vi "HW_Server.vi"(8 "Error In":errorcluster) -> (0 "Error Out":errorcluster)   [LabVIEW 2011]
doc: "This VI will handle communication with Main VI and HW."
uses:
  Controls/TransparencyEffectOperations.ctl
  Controls/Global Stop - Operations.ctl
panel:
  # "HW SERVER"
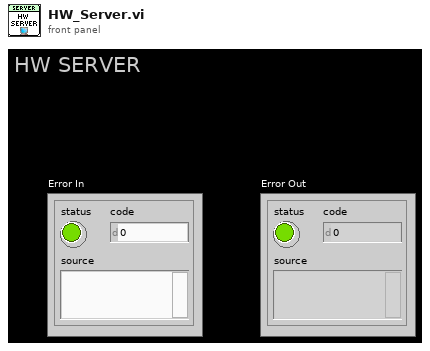
[diagram p1: front panel]
types:
  T1 = typedef "TransparencyEffectOperations.ctl" = enum16{"Show", "Hide 80%", "Hide All"}
  T2 = typedef "Global Stop - Operations.ctl" = enum16{"Stop", "Status", "Init"}
  T3 = typedef "HW Server Status.ctl" = enum16{"NO CHASSIS", "NO MODULES", "OK"}
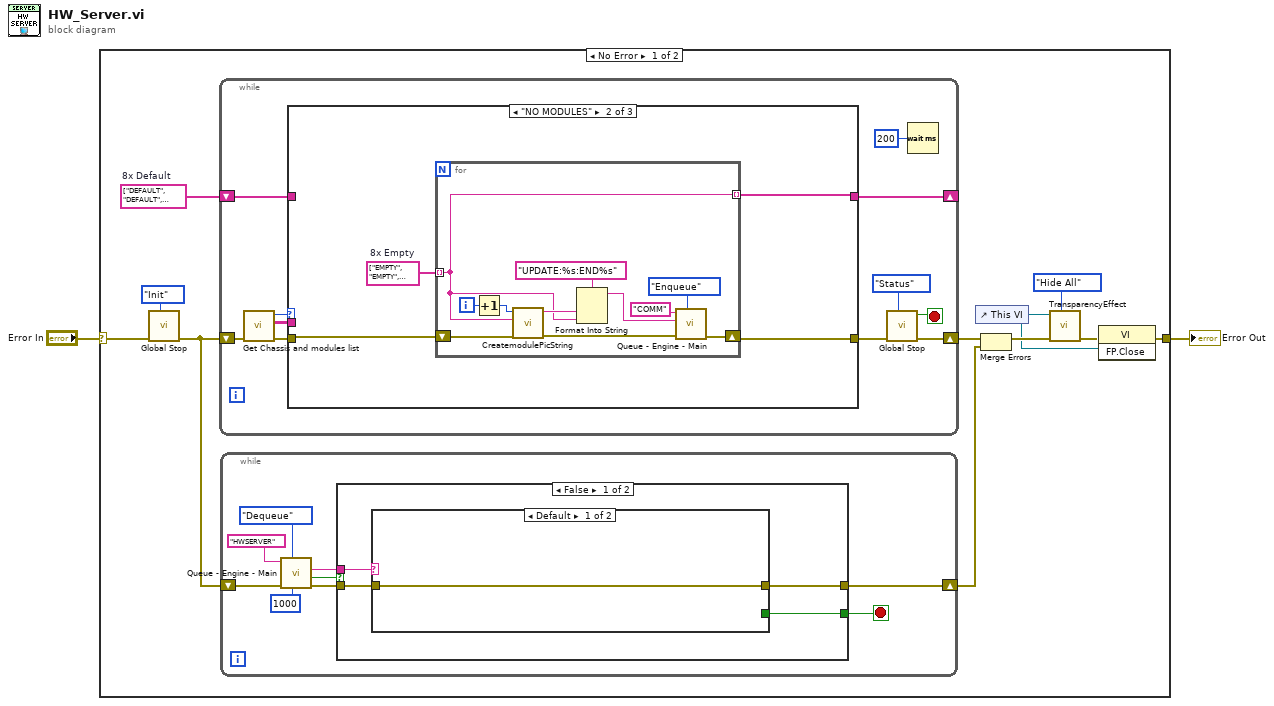
[diagram p0: block diagram]
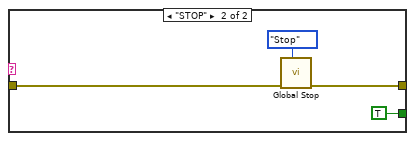
[diagram p2: hidden frame]
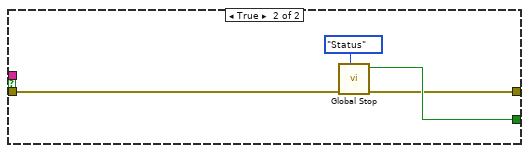
[diagram p3: hidden frame]
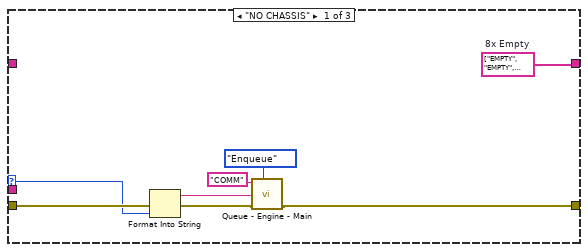
[diagram p4: hidden frame]
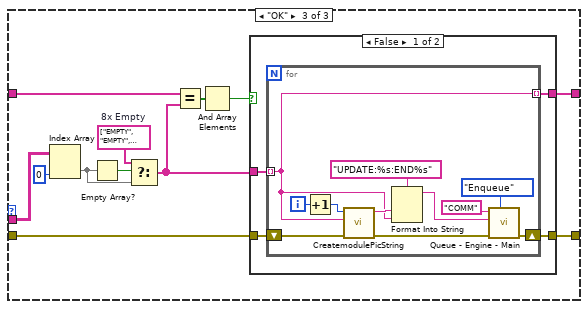
[diagram p5: hidden frame]
diagram:
  n1 = case shown="No Error" "Error In" {
    selector: "Error In" -> [w10 w99]
    tunnel: [w4 w99] -> w2
    frame No Error {
      w13 = string[] ["DEFAULT", "DEFAULT", "DEFAULT", "DEFAULT", "DEFAULT", "DEFAULT", "DEFAULT", "DEFAULT"]  # 8x Default
      n2 = call "Global Stop.vi"("Operation"=Global_Stop_-_Operations."Init", "error in (no error)"=w10) -> ("error out"=w3:errorcluster)  [unwired: 8 in, 1 out]
      n3 = while {
        shift-right: [w39] -> w11
        shift-left: w3 -> [w45]
        shift-right: [w42] -> _
        shift-left: w13 -> [w43]
        stop <- w38 stop-if-true
        n4 = call "Get Chassis and modules list.vi"("error in"=w45) -> ("error out"=w41:errorcluster, "Modules Out"=w44:string[][], "Status Out"=w36:T3)  [unwired: 8 in]
        n5 = case shown="\"NO MODULES\"" w36 {
          selector: w36 -> [w52 _ _]
          tunnel: w44 -> [_ _ w80]
          tunnel: w43 -> [_ _ w79]
          tunnel: [w54 w55 w72] -> w42
          tunnel: w41 -> [w53 w57 w71]
          tunnel: [w48 w56 w70] -> w40
          frame "NO CHASSIS" {
            w54 = string[] ["EMPTY", "EMPTY", "EMPTY", "EMPTY", "EMPTY", "EMPTY", "EMPTY", "EMPTY"]  # 8x Empty
            n6 = Format Into String(error in=w53, w52) -> (resulting string=w47:string, error out=w49:errorcluster)  [unwired: 2 in]
            n7 = call "Queue - Engine - Main.vi"("Operation"=enum16{"Enqueue", "Dequeue", "Flush", "Release"}."Enqueue", "error in"=w49, "Queue Data In"=w47, "Queue Name In"="COMM") -> ("error out"=w48:errorcluster)  [unwired: 5 in, 2 out]
          }
          frame "NO MODULES" {
            w58 = string[] ["EMPTY", "EMPTY", "EMPTY", "EMPTY", "EMPTY", "EMPTY", "EMPTY", "EMPTY"]  # 8x Empty
            n8 = for {
              tunnel: w58 -> [w64] mode=indexing
              shift-right: [w62] -> w56
              shift-left: w57 -> [w65]
              tunnel: [w64] -> w55 mode=indexing
              i -> [w69]
              n9 = Increment(x=w69) -> (x+1=w68:i32)
              n10 = call "CreatemodulePicString.vi"("Error In"=w65, "input string"=w64, "Slot Nr"=w68) -> ("Error Out"=w63:errorcluster, "Pic String Out"=w66:string)  [unwired: 7 in]
              n11 = Format Into String(format string="UPDATE:%s:END%s", w66, w64) -> (resulting string=w61:string)  [unwired: 2 in, 1 out]
              n12 = call "Queue - Engine - Main.vi"("Operation"=enum16{"Enqueue", "Dequeue", "Flush", "Release"}."Enqueue", "error in"=w63, "Queue Data In"=w61, "Queue Name In"="COMM") -> ("error out"=w62:errorcluster)  [unwired: 5 in, 2 out]
            }
          }
          frame "OK" {
            w76 = string[] ["EMPTY", "EMPTY", "EMPTY", "EMPTY", "EMPTY", "EMPTY", "EMPTY", "EMPTY"]  # 8x Empty
            n13 = Index Array(array=w80, index (col)=0 ("disabled index (col)")) -> (element=w74:string[])  [unwired: 1 in]
            n14 = Empty Array?(array=w74) -> (empty?=w77:bool)
            n15 = Select(t=w76, s=w77, f=w74) -> (s? t:f=w73:string[])
            n16 = Equal?(x=w79, y=w73) -> (x = y?=w75:bool[])
            n17 = And Array Elements(Boolean array=w75) -> (logical AND=w78:bool)
            n18 = case shown="False" w78 {
              tunnel: w73 -> [w85 w98]
              tunnel: [w84 w97] -> w70
              tunnel: [w83 w98] -> w72
              tunnel: w71 -> [w82 w97]
              frame False {
                n19 = for {
                  tunnel: w85 -> [w91] mode=indexing
                  shift-right: [w87] -> w84
                  shift-left: w82 -> [w92]
                  tunnel: [w91] -> w83 mode=indexing
                  i -> [w96]
                  n20 = Increment(x=w96) -> (x+1=w95:i32)
                  n21 = call "CreatemodulePicString.vi"("Error In"=w92, "input string"=w91, "Slot Nr"=w95) -> ("Error Out"=w88:errorcluster, "Pic String Out"=w93:string)  [unwired: 7 in]
                  n22 = Format Into String(format string="UPDATE:%s:END%s", w93, w91) -> (resulting string=w86:string)  [unwired: 2 in, 1 out]
                  n23 = call "Queue - Engine - Main.vi"("Operation"=enum16{"Enqueue", "Dequeue", "Flush", "Release"}."Enqueue", "error in"=w88, "Queue Data In"=w86, "Queue Name In"="COMM") -> ("error out"=w87:errorcluster)  [unwired: 5 in, 2 out]
                }
              }
              frame True {
              }
            }
          }
        }
        n24 = call "Global Stop.vi"("Operation"=Global_Stop_-_Operations."Status", "error in (no error)"=w40) -> ("error out"=w39:errorcluster, "Stop?"=w38:bool)  [unwired: 8 in]
        n25 = Wait (ms)(milliseconds to wait=u32 200) -> ()  [unwired: 1 out]
      }
      n26 = while {
        shift-right: [w21] -> w12
        shift-left: w3 -> [w19]
        stop <- w22 stop-if-true
        n27 = call "Queue - Engine - Main.vi"("timeout in ms (-1)"=1000, "Operation"=enum16{"Enqueue", "Dequeue", "Flush", "Release"}."Dequeue", "error in"=w19, "Queue Name In"="HWSERVER" ("name")) -> ("error out"=w20:errorcluster, "timed out?"=w14:bool, "Data Out"=w15:string)  [unwired: 5 in]
        n28 = case shown="False" w14 {
          tunnel: w20 -> [w26 w33]
          tunnel: [w25 w32] -> w21
          tunnel: [w24 w34] -> w22
          tunnel: w15 -> [w23 _]
          frame False {
            n29 = case shown="Default" w23 {
              tunnel: w26 -> [w27 w30]
              tunnel: [w27 w29] -> w25
              tunnel: [_ TRUE] -> w24
              frame Default {
              }
              frame "STOP" {
                n30 = call "Global Stop.vi"("Operation"=Global_Stop_-_Operations."Stop", "error in (no error)"=w30) -> ("error out"=w29:errorcluster)  [unwired: 8 in, 1 out]
              }
            }
          }
          frame True {
            n31 = call "Global Stop.vi"("Operation"=Global_Stop_-_Operations."Status", "error in (no error)"=w33) -> ("error out"=w32:errorcluster, "Stop?"=w34:bool)  [unwired: 8 in]
          }
        }
      }
      n32 = control-ref of="This VI"() -> (w6:refnum<vi>)
      n33 = Merge Errors(w11, w12) -> (w7:errorcluster)
      n34 = call "TransparencyEffect.vi"("Operation"=TransparencyEffectOperations."Hide All", "error in"=w7, "VI Ref in"=w6) -> ("error out"=w5:errorcluster)  [unwired: 8 in]
      n35 = invoke class="VI" method="FP.Close"(reference=w6, error in=w5) -> (error out=w4:errorcluster)  [unwired: 1 in, 2 out]
    }
    frame Error {
    }
  }
  "Error Out" <- w2
